vi "POP_CtlRect.vi"(8 "Error In":errorcluster, 10 "CtlRef":refnum<vi>, 11 "PopupRef":refnum<vi>) -> (0 "Error Out":errorcluster, 1 "Panes?":bool, 2 "Pane Refnum":refnum<vi>, 3 "CtrlRect":T1)   [LabVIEW 2016]
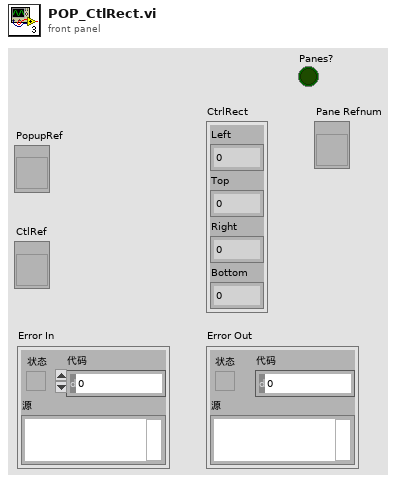
[diagram p1: front panel]
types:
  T1 = cluster{"Left":i32, "Top":i32, "Right":i32, "Bottom":i32}
  T2 = typedef "LVPositionTypeDef.ctl" = cluster{"Left":i32, "Top":i32}
  T3 = typedef "LVBoundsTypeDef.ctl" = cluster{"Width":u32, "Height":u32}
  T4 = typedef "LVPointTypeDef.ctl" = cluster{"Horizontal":i16, "Vertical":i16}
  T5 = cluster{"Horizontal":i32, "Vertical":i32, i32, i32}
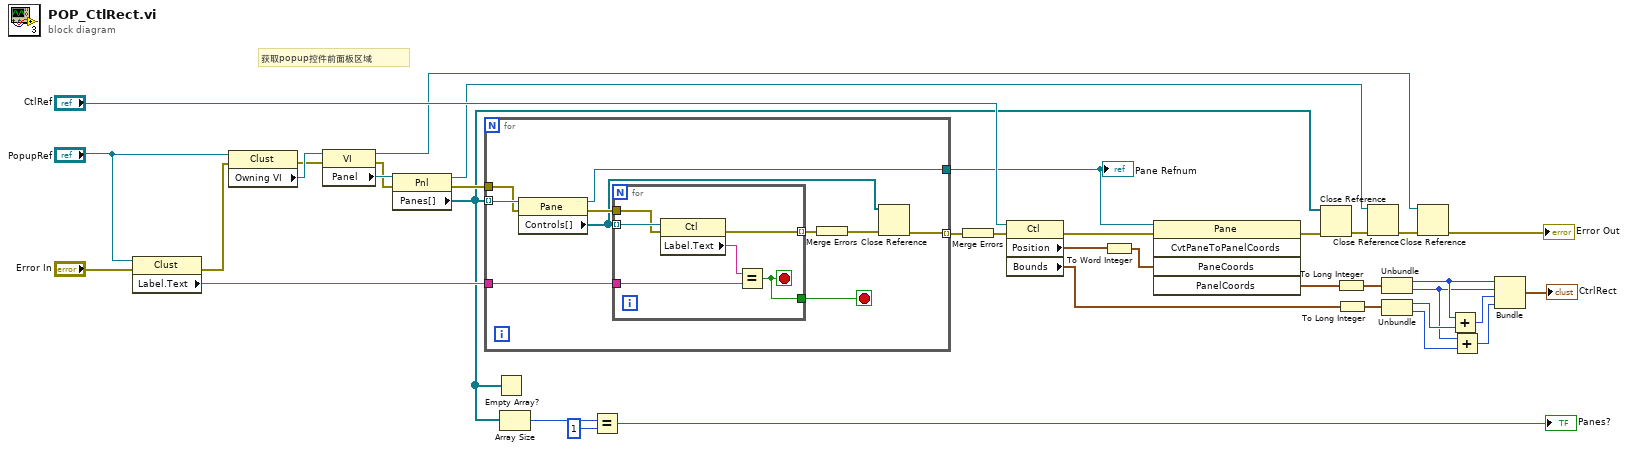
[diagram p0: block diagram]
diagram:
  # "获取popup控件前面板区域"
  n1 = property class="Clust"(reference="PopupRef", error in="Error In") -> (error out=w32:errorcluster, "Label.Text"=w31:string)  [unwired: 1 out]
  n2 = property class="Clust"(reference="PopupRef", error in=w32) -> (error out=w34:errorcluster, "Owning VI"=w35:refnum<vi>)  [unwired: 1 out]
  n3 = property class="VI"(reference=w35, error in=w34) -> (reference out=w12:refnum<vi>, error out=w36:errorcluster, "Panel"=w37:refnum<vi>)
  n4 = property class="Pnl"(reference=w37, error in=w36) -> (reference out=w13:refnum<vi>, error out=w30:errorcluster, "Panes[]"=w4:refnum<vi>[])
  n5 = for {
    tunnel: w4 -> [w47] mode=indexing
    tunnel: w31 -> [w44]
    tunnel: w30 -> [w46]
    tunnel: [w43] -> w25
    tunnel: [w38] -> w28 mode=indexing
    stop <- w42 stop-if-true
    n6 = property class="Pane"(reference=w47, error in=w46) -> (reference out=w43:refnum<vi>, error out=w45:errorcluster, "Controls[]"=w39:refnum<vi>[])
    n7 = for {
      tunnel: w39 -> [w53] mode=indexing
      tunnel: w45 -> [w52]
      tunnel: w44 -> [w51]
      tunnel: [w49] -> w42
      tunnel: [w48] -> w41 mode=indexing
      stop <- w49 stop-if-true
      n8 = property class="Ctl"(reference=w53, error in=w52) -> (error out=w48:errorcluster, "Label.Text"=w50:string)  [unwired: 1 out]
      n9 = Equal?(x=w50, y=w51) -> (x = y?=w49:bool)
    }
    n10 = Merge Errors(w41) -> (w40:errorcluster)
    n11 = Close Reference(reference=w39, error in (no error)=w40) -> (error out=w38:errorcluster)
  }
  "Pane Refnum" <- w25
  n12 = Empty Array?(array=w4) -> ()  [unwired: 1 out]
  n13 = Array Size(array=w4) -> (size(s)=w3:i32)
  n14 = Equal?(x=w3, y=1) -> (x = y?=→"Panes?":bool)
  n15 = Merge Errors(w28) -> (w24:errorcluster)
  n16 = property class="Ctl"(reference="CtlRef", error in=w24) -> (error out=w23:errorcluster, "Position"=w6:T2, "Bounds"=w17:T3)  [unwired: 1 out]
  n17 = To Word Integer(number=w6) -> (16bit integer=w19:cluster{"Left":i16, "Top":i16})
  n18 = invoke class="Pane" method="CvtPaneToPanelCoords"(reference=w25, error in=w23, "PaneCoords"=w19) -> (error out=w14:errorcluster, "PanelCoords"=w5:T4)  [unwired: 2 in, 3 out]
  n19 = Close Reference(reference=w4, error in (no error)=w14) -> (error out=w8:errorcluster)
  n20 = To Long Integer(number=w5) -> (32bit integer=w18:cluster{"Horizontal":i32, "Vertical":i32})
  n21 = To Long Integer(number=w17) -> (32bit integer=w16:cluster{"Width":i32, "Height":i32})
  n22 = Close Reference(reference=w13, error in (no error)=w8) -> (error out=w7:errorcluster)
  n23 = Unbundle(w18) -> ("Horizontal"=w27:i32, "Vertical"=w21:i32)
  n24 = Unbundle(w16) -> ("Width"=w26:i32, "Height"=w15:i32)
  n25 = Close Reference(reference=w12, error in (no error)=w7) -> (error out=→"Error Out":errorcluster)
  n26 = Add(x=w27, y=w26) -> (x+y=w22:i32)
  n27 = Add(x=w21, y=w15) -> (x+y=w20:i32)
  n28 = Bundle("Horizontal"=w27, "Vertical"=w21, w22, w20) -> (→"CtrlRect":T5)  [unwired: 1 in]
